vi "MicroStrain 3DM-GXx Continuous Mode.vi"() -> ()   [LabVIEW 2012]
doc: "This VI demonstrates the procedure for using the device in continuous (streaming) measurement mode."
uses:
  <instrlib>/MicroStrain 3DM-GXx/Public/Data/Parse Message VIs/Parse (Euler Angles).vi
  <instrlib>/MicroStrain 3DM-GXx/Public/Data/Parse Message VIs/Parse (Delta Values).vi
  <instrlib>/MicroStrain 3DM-GXx/Public/Data/Parse Message VIs/Parse (Orientation Matrix).vi
  <instrlib>/MicroStrain 3DM-GXx/Public/Data/Parse Message VIs/Parse (Orientation Update Matrix).vi
  <instrlib>/MicroStrain 3DM-GXx/Public/Data/Parse Message VIs/Parse (Internal Device Temperature).vi
  <instrlib>/MicroStrain 3DM-GXx/Public/Data/Parse Message VIs/Parse (Acceleration, Angular Rate, And Magnetometer Vectors).vi
  <instrlib>/MicroStrain 3DM-GXx/Public/Data/Parse Message VIs/Parse (Gyro Stabilized Acceleration, Angular Rate, And Magnetometer Vectors).vi
  <instrlib>/MicroStrain 3DM-GXx/Public/Data/Parse Message VIs/Parse (Raw Acceleration And Angular Rates).vi
  <instrlib>/MicroStrain 3DM-GXx/MicroStrain 3DM-GXx.lvlib
panel:
  out "Measurements":T1(tab)
  out "Raw Vector Timer":u32
  out "Raw Angular Rate Vector":sgl[](array[numeric])
  out "Raw Accelerometer Vector":sgl[](array[numeric])
  out "Delta Timer":u32
  out "Delta Velocity Vector":sgl[](array[numeric])
  out "Delta Angle Vector":sgl[](array[numeric])
  out "Orientation Matrix Timer":u32
  out "Orientation Matrix":sgl[][](array[numeric])
  out "Orientation Update Matrix Timer":u32
  out "Orientation Update Matrix":sgl[][](array[numeric])
  out "AAM Timer":u32
  out "Angular Rate":sgl[](array[numeric])
  out "Acceleration":sgl[](array[numeric])
  out "Magnetometer Vector":sgl[](array[numeric])
  out "Euler Timer":u32
  out "Yaw":sgl
  out "Pitch":sgl
  out "Roll":sgl
  out "Timer":u32
  out "Temperature":sgl
  out "GS AAM Timer":u32
  out "Gyro Stabilized Magnetometer Vetor":sgl[](array[numeric])
  out "Gyro Stabilized Angular Rate Vector":sgl[](array[numeric])
  out "Gyro Stabilized Acceleration Vector":sgl[](array[numeric])
  in  "VISA resource name":refnum<visa-resource-name>
  in  "Continuous Measurement Type":u16(ring)=5 items=["Euler Angles"=5, "DeltaAngle & DeltaVelocity"=1, "Orientation Matrix"=2, "Orientation Update Matrix"=3, "Acceleration, Angular Rate & Magnetometer Vectors"=4, "Gyro Stabilized Acceleration, Angular Rate & Magnetometer"=7, "Temperatures"=6, "Raw Accelerometer and Angular Rate"=0]
  in  "Sample Rate (100 Hz)":u16=100 min=1 max=300
  in  "Stop Continuous Measurement":bool
  # "(c) 2009 - 2011 National Instruments.  ALL RIGHTS RESERVED."
  # "This VI demonstrates the procedure for using the device in continuous (streaming) measurement mode.  The user is able to select the \ncontinuous measurement type before running the VI.  To change the continuous measurement type the device must be brought out \nof continuous mode, then continuous mode must be re-initialized with the new measurement type.  This can be accomplished by \npressing the stop button, choosing a new continuous measurement type and then running the VI."
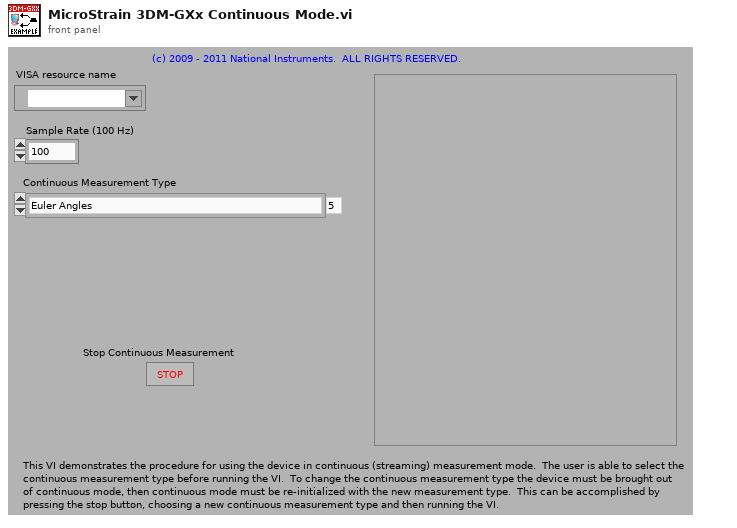
[diagram p1: front panel]
types:
  T1 = enum32{"Raw Accelerometer and Angular Rate", "Delta Angle and Delta Velocity", "Orientation Matrix", "Orientation Update Matrix", "Acceleration, Angular Rate & Magnetometer Vectors", "Euler Angles", "Temperatures", "Gyro Stabilized Acceleration, Angular Rate & Magnetometer"}
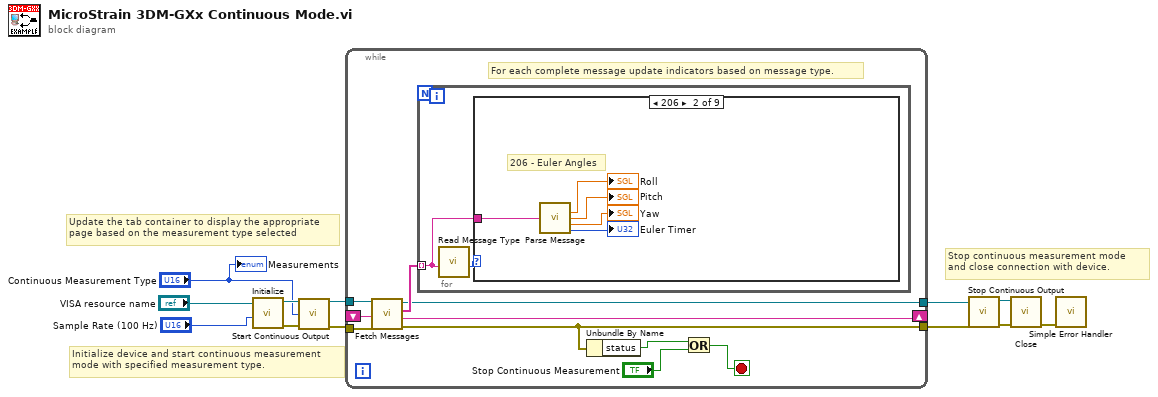
[diagram p0: block diagram]
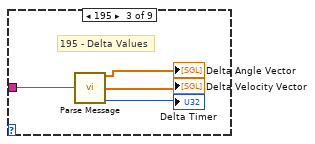
[diagram p3: hidden frame]
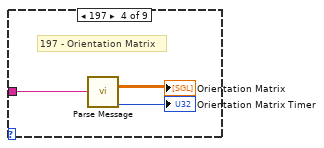
[diagram p4: hidden frame]
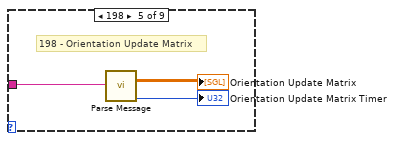
[diagram p5: hidden frame]
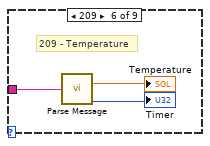
[diagram p6: hidden frame]
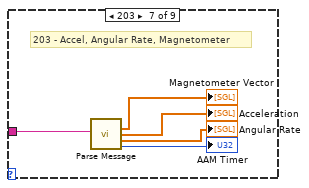
[diagram p7: hidden frame]
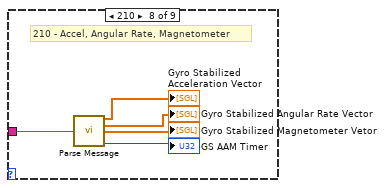
[diagram p8: hidden frame]
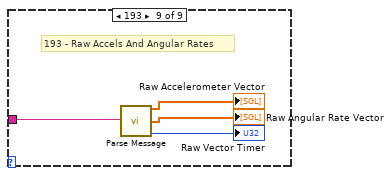
[diagram p9: hidden frame]
diagram:
  # "Update the tab container to display the appropriate\npage based on the measurement type selected"
  # "Stop continuous measurement mode \nand close connection with device."
  # "Initialize device and start continuous measurement \nmode with specified measurement type."
  n1 = call <instrlib>:"Initialize.vi"("Sample Rate (100 Hz)"="Sample Rate (100 Hz)", "VISA resource name"="VISA resource name") -> ("error out"=w11:errorcluster, "VISA resource name out"=w12:refnum<visa-resource-name>)  [unwired: 8 in]
  n2 = call <instrlib>:"Start Continuous Output.vi"("VISA resource name"=w12, "Continuous Measurement Type (Raw Accelerometer and Angular Rate)"="Continuous Measurement Type", "error in (no error)"=w11) -> ("VISA resource name out"=w8:refnum<visa-resource-name>, "error out"=w7:errorcluster)  [unwired: 11 in]
  n3 = while {
    tunnel: w8 -> [w22]
    tunnel: w7 -> [w21]
    shift-right: [w19] -> _
    shift-left: _ -> [w20]
    tunnel: [w16] -> w2
    tunnel: [w17] -> w3
    stop <- w13 stop-if-true
    # "For each complete message update indicators based on message type."
    n4 = call <instrlib>:"Fetch Messages.vi"("error in (no error)"=w21, "Remainder In"=w20, "VISA resource name"=w22) -> ("error out"=w16:errorcluster, "Remainder Out"=w19:string, "Complete Messages"=w18:string[], "VISA resource name out"=w17:refnum<visa-resource-name>)  [unwired: 5 in]
    n5 = for {
      tunnel: w18 -> [w24] mode=indexing
      n6 = call <instrlib>:"Read Message Type.vi"("Message"=w24) -> ("Ring"=w23:u16)  [unwired: 10 in]
      n7 = case shown="206" w23 {
        tunnel: w24 -> [_ w29 w33 w36 w39 w42 w47 w52 w56]
        frame 0, Default {
          # "Unknown message type. \nDisregard message."
        }
        frame 206 {
          # "206 - Euler Angles"
          n8 = call-poly <instrlib>:"Parse Message.vi"("Message In"=w29) -> ("Roll"=→"Roll":sgl, "Pitch"=→"Pitch":sgl, "Yaw"=→"Yaw":sgl, "Timer"=→"Euler Timer":u32)  [unwired: 11 in]
        }
        frame 195 {
          # "195 - Delta Values"
          n9 = call-poly <instrlib>:"Parse Message.vi"("Message In"=w33) -> ("DeltaAngleVector"=→"Delta Angle Vector":sgl[], "DeltaVelocityVector"=→"Delta Velocity Vector":sgl[], "Timer"=→"Delta Timer":u32)  [unwired: 12 in]
        }
        frame 197 {
          # "197 - Orientation Matrix"
          n10 = call-poly <instrlib>:"Parse Message.vi"("Message In"=w36) -> ("Orientation Matrix"=→"Orientation Matrix":sgl[][], "Timer"=→"Orientation Matrix Timer":u32)  [unwired: 13 in]
        }
        frame 198 {
          # "198 - Orientation Update Matrix"
          n11 = call-poly <instrlib>:"Parse Message.vi"("Message In"=w39) -> ("Orientation Update Matrix"=→"Orientation Update Matrix":sgl[][], "Timer"=→"Orientation Update Matrix Timer":u32)  [unwired: 13 in]
        }
        frame 209 {
          # "209 - Temperature"
          n12 = call-poly <instrlib>:"Parse Message.vi"("Message In"=w42) -> ("Temperature"=→"Temperature":sgl, "Timer"=→"Timer":u32)  [unwired: 13 in]
        }
        frame 203 {
          # "203 - Accel, Angular Rate, Magnetometer"
          n13 = call-poly <instrlib>:"Parse Message.vi"("Message In"=w47) -> ("Magnetometer Vector"=→"Magnetometer Vector":sgl[], "Acceleration"=→"Acceleration":sgl[], "Angular Rate"=→"Angular Rate":sgl[], "Timer"=→"AAM Timer":u32)  [unwired: 11 in]
        }
        frame 210 {
          # "210 - Accel, Angular Rate, Magnetometer"
          n14 = call-poly <instrlib>:"Parse Message.vi"("Message In"=w52) -> ("Gyro Stabilized Acceleration Vector"=→"Gyro Stabilized Acceleration Vector":sgl[], "Gyro Stabilized Angular Rate Vector"=→"Gyro Stabilized Angular Rate Vector":sgl[], "Gyro Stabilized Magnetometer Vetor"=→"Gyro Stabilized Magnetometer Vetor":sgl[], "Timer"=→"GS AAM Timer":u32)  [unwired: 11 in]
        }
        frame 193 {
          # "193 - Raw Accels And Angular Rates"
          n15 = call-poly <instrlib>:"Parse Message.vi"("Message In"=w56) -> ("Raw Accelerometer Vector"=→"Raw Accelerometer Vector":sgl[], "Raw Angular Rate Vector"=→"Raw Angular Rate Vector":sgl[], "Timer"=→"Raw Vector Timer":u32)  [unwired: 12 in]
        }
      }
    }
    n16 = Unbundle By Name(w16) -> ("status"=w14:bool)
    n17 = Or(x=w14, y="Stop Continuous Measurement") -> (x .or. y?=w13:bool)
  }
  n18 = call <instrlib>:"Stop Continuous Output.vi"("error in (no error)"=w2, "VISA resource name"=w3) -> ("error out"=w6:errorcluster, "VISA resource name out"=w5:refnum<visa-resource-name>)  [unwired: 8 in]
  n19 = call <instrlib>:"Close.vi"("error in (no error)"=w6, "VISA resource name"=w5) -> ("error out"=w4:errorcluster)  [unwired: 9 in]
  n20 = call <vilib>:"Simple Error Handler.vi"("error in (no error)"=w4) -> ()  [unwired: 4 in, 5 out]
  "Measurements" <- "Continuous Measurement Type"
